vi "FTW-Messenger-WaitForInit.vi"(0 "Messenger":refnum<class "FTW-Messenger.lvclass">, 5 "Expected Response":variant, 7 "Timeout (500msec)":i32=500, 11 "error in":errorcluster) -> (4 "Initialized Messenger":refnum<class "FTW-Messenger.lvclass">, 6 "Response":variant, 8 "Timed out?":bool, 15 "error out":errorcluster)   [LabVIEW 2013, in "FTW-Messenger.lvclass"]
uses:
  FTW-Messenger.lvclass
  FTW-Messenger.lvclass/FTW-Messenger.ctl
  Container/FTW-Container.lvclass
panel:
  # "Inputs"
  # "Outputs"
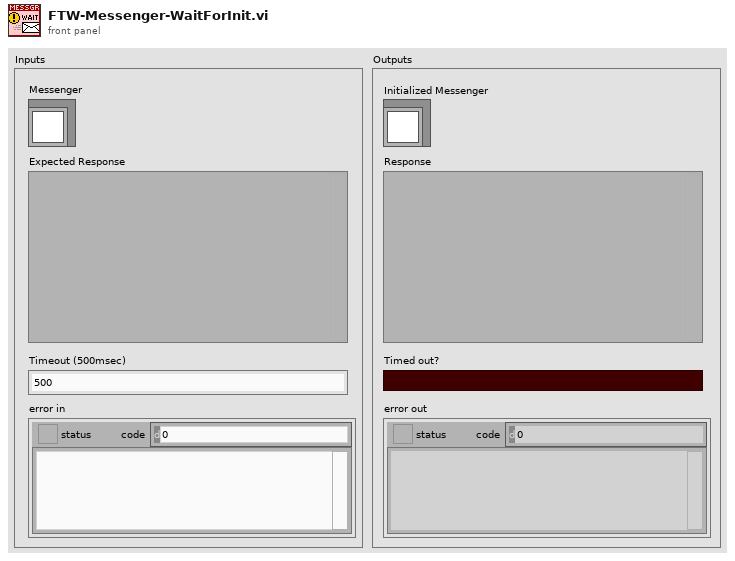
[diagram p1: front panel]
types:
  T1 = cluster{"Response":refnum<class "FTW-Container.lvclass">, "Messenger":refnum<class>}
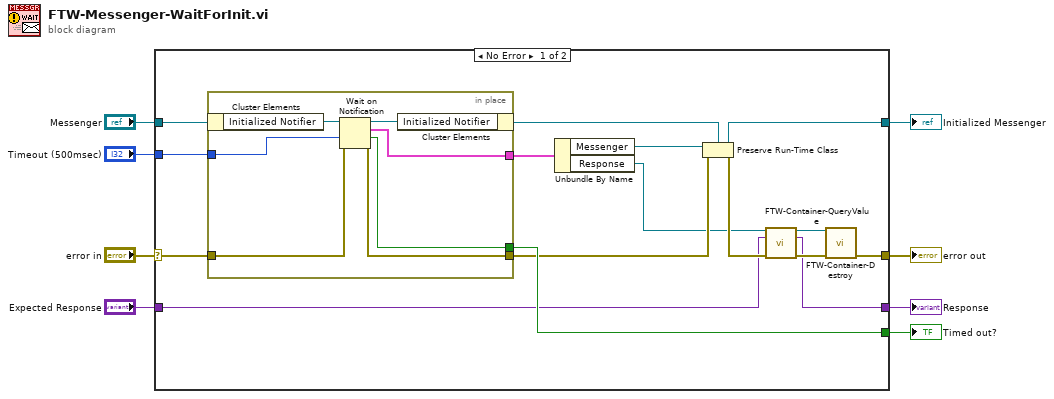
[diagram p0: block diagram]
diagram:
  n1 = case shown="No Error" "error in" {
    selector: "error in" -> [w24 w34]
    tunnel: [w13 w34] -> w6
    tunnel: [w20 w33] -> w7
    tunnel: "Messenger" -> [w10 w33]
    tunnel: "Timeout (500msec)" -> [w23 _]
    tunnel: [w21 _] -> w3
    tunnel: [w15 w32] -> w2
    tunnel: "Expected Response" -> [w11 w32]
    frame No Error {
      n2 = in-place {
        in-place-border: w24 -> [w31]
        in-place-border: w23 -> [w30]
        in-place-border: [w29] -> w22
        in-place-border: [w28] -> w21
        in-place-border: [w27] -> w19
        n3 = in-place-cluster #1(w10) -> ("Initialized Notifier"=w26:refnum<notifier>)
        n4 = Wait on Notification(notifier=w26, timeout in ms (-1)=w30, error in (no error)=w31) -> (notifier out=w25:refnum<notifier>, notification=w29:T1, timed out?=w28:bool, error out=w27:errorcluster)  [unwired: 1 in]
        n5 = in-place-cluster #1("Initialized Notifier"=w25) -> (w9:refnum<class "FTW-Messenger.lvclass">)
      }
      n6 = Unbundle By Name(w22) -> ("Messenger"=w18:refnum<class>, "Response"=w12:refnum<class "FTW-Container.lvclass">)
      n7 = Preserve Run-Time Class(object in=w18, error in=w19, 2:w9) -> (object out=w20:refnum<class "FTW-Messenger.lvclass">, error out=w14:errorcluster)
      n8 = call "FTW-Container-QueryValue.vi"("Container"=w12, "Type and Defaults"=w11, "error in"=w14) -> ("Container out"=w17:refnum<class "FTW-Container.lvclass">, "Result"=w15:variant, "error out"=w16:errorcluster)  [unwired: 10 in]
      n9 = call "FTW-Container-Destroy.vi"("Container"=w17, "error in"=w16) -> ("error out"=w13:errorcluster)  [unwired: 13 in]
    }
    frame Error {
    }
  }
  "Initialized Messenger" <- w7
  "error out" <- w6
  "Timed out?" <- w3
  "Response" <- w2
